vi "ITX Example.vi"() -> ()   [LabVIEW 2013]
panel:
  in  "number4":dbl=7.0
  in  "number3":dbl=5.0
  in  "number2":dbl=3.0
  in  "number1":dbl
  in  "plot2":cluster{dbl[], dbl[]}(graph)={[100000.0, 125892.54117941661, 158489.3192461114, 199526.2314968879, 251188.6431509582, 316227.7660168379, 398107.1705534969, 501187.2336272725, 630957.344480193, 794328.2347242822, 1000000.0, 1258925.411794166, 1584893.192461114, 1995262.314968879, 2511886.431509582, 3162277.66016838, 3981071.705534969, 5011872.336272725, 6309573.44480193, 7943282.347242822, 10000000.0, 12589254.117941663, 15848931.924611142, 19952623.14968883, 25118864.315095823, 31622776.60168379, 39810717.05534969, 50118723.36272725, 63095734.44801943, 79432823.47242822, 100000000.0, 125892541.17941661, 158489319.2461111, 199526231.49688828, 251188643.1509582, 316227766.01683795, 398107170.5534969, 501187233.6272715, 630957344.4801943, 794328234.7242821, 1000000000.0], [0.0604667, 0.002433367000000003, 0.02919999, 0.036766673, 0.07459995999999999, 0.058766570000000004, 0.02630003, -0.0314666, 0.03733326, -0.01006674, 0.005166649999999999, -0.013299987000000001, 0.01406666, 0.008233343, 0.008333337, -0.003000007000000001, 0.00923335, 0.009000003, 0.011999996700000001, 0.012433329, 0.0049, 0.007766663, 0.009300005, 0.0045000027, 0.006500002, 0.008566672000000001, 0.0043333317, 0.002000004, 0.005333332, 0.0038999987, 0.003166668, 0.001799999, 0.0021333357, 0.001133332, 0.004933332, 0.0021333317, 0.0025000014, 0.004033335, 0.0020666647, 0.002000003, 0.001433333]}
  in  "plot1":cluster{dbl[], dbl[]}(graph)={[100000.0, 125892.54117941661, 158489.3192461114, 199526.2314968879, 251188.6431509582, 316227.7660168379, 398107.1705534969, 501187.2336272725, 630957.344480193, 794328.2347242822, 1000000.0, 1258925.411794166, 1584893.192461114, 1995262.314968879, 2511886.431509582, 3162277.66016838, 3981071.705534969, 5011872.336272725, 6309573.44480193, 7943282.347242822, 10000000.0, 12589254.117941663, 15848931.924611142, 19952623.14968883, 25118864.315095823, 31622776.60168379, 39810717.05534969, 50118723.36272725, 63095734.44801943, 79432823.47242822, 100000000.0, 125892541.17941661, 158489319.2461111, 199526231.49688828, 251188643.1509582, 316227766.01683795, 398107170.5534969, 501187233.6272715, 630957344.4801943, 794328234.7242821, 1000000000.0], [0.002666666, 0.004400004, 0.0028333406, 0.005400007, -6.666699999999994e-05, 0.006833331, 0.001999997, 0.003966663, 0.003200001, 0.003733337, 0.0034666673, 0.007700011, 0.006166671, 0.004900002000000001, 0.004133333, 0.006633334, 0.01919998, 0.06286665999999999, 0.12583327, 0.2032, 0.2774667, 0.3839666, 0.4441999, 0.4771333, 0.5964335, 0.6360335, 0.6610668000000001, 0.6360334, 0.6508001, 0.6097, 0.5689667, 0.5584333, 0.5266666, 0.4415334, 0.39940000000000003, 0.2484999, 0.3907333, 0.2028, 0.4827999, 0.3610667, 0.3846001]}
  in  "plot0":cluster{dbl[], dbl[]}(graph)={[100000.0, 125892.54117941661, 158489.3192461114, 199526.2314968879, 251188.6431509582, 316227.7660168379, 398107.1705534969, 501187.2336272725, 630957.344480193, 794328.2347242822, 1000000.0, 1258925.411794166, 1584893.192461114, 1995262.314968879, 2511886.431509582, 3162277.66016838, 3981071.705534969, 5011872.336272725, 6309573.44480193, 7943282.347242822, 10000000.0, 12589254.117941663, 15848931.924611142, 19952623.14968883, 25118864.315095823, 31622776.60168379, 39810717.05534969, 50118723.36272725, 63095734.44801943, 79432823.47242822, 100000000.0, 125892541.17941661, 158489319.2461111, 199526231.49688828, 251188643.1509582, 316227766.01683795, 398107170.5534969, 501187233.6272715, 630957344.4801943, 794328234.7242821, 1000000000.0], [3.929161e-11, 2.28883e-11, 7.743881e-11, 1.83106e-10, 2.9793e-10, 3.948231e-10, 4.566212e-10, 4.592915e-10, 4.261035e-10, 4.1885560000000003e-10, 3.776569e-10, 4.1008169999999997e-10, 3.9406009999999996e-10, 3.677387e-10, 3.864308e-10, 4.043599e-10, 4.2495899999999994e-10, 4.837062e-10, 4.768397e-10, 4.913361e-10, 4.779835e-10, 4.226704e-10, 3.98256e-10, 6.107368e-10, 8.262671999999999e-10, 1.922619e-09, 1.959242e-09, 1.733406e-09, 1.485832e-09, 1.0738448e-09, 1.396568e-09, 2.188124e-09, 3.49428e-10, 2.4109e-10, 3.1395149999999995e-10, 2.441421e-10, 8.049056999999999e-11, 4.3487779999999995e-11, 9.269760999999999e-11, 2.136242e-11, 1.90736e-11]}
  in  "Notes":string="date and time are AUTOMATICALLY saved!\nwrite your experiment notes here"
  in  "path":path=path "C:/Users/voodoo.SEAGATE/Desktop/datatest"
  in  "filename":string="datatest"
  in  "wavenames (.Vx, etc)":string[](array[string])=["plot0", "plot1", "plot2", "number1", "number2", "number3", "number4"]
  # "give everything you are saving a name,\nor else you will become confused!"
  # "\"basic\" data format is XY graph:"
  # "\"numbers\" can be saved too:"
  # "just do this to make \"XY graphs\" out of them:"
  # "make array of graphs\nto save them all:"
  # "- set path to folder\n- set base filename\n   (up to 999,999 files with same base name \n    an be written in one folder)\n- type some comments"
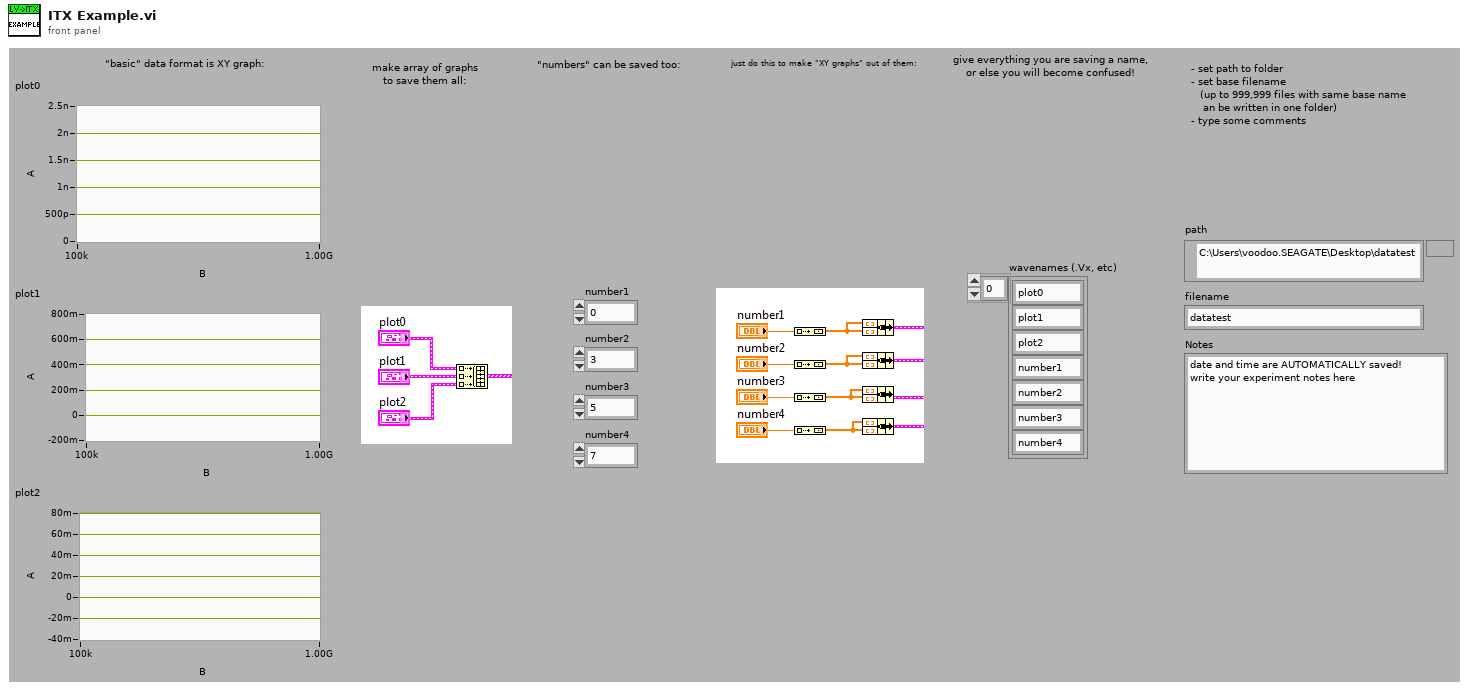
[diagram p1: front panel]
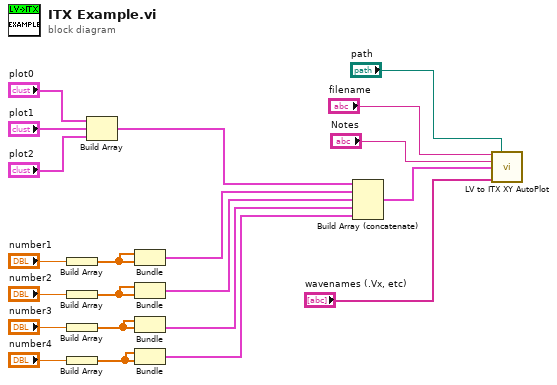
[diagram p0: block diagram]
diagram:
  n1 = Build Array("number1") -> (w15:dbl[])
  n2 = Build Array("number2") -> (w11:dbl[])
  n3 = Build Array("number3") -> (w10:dbl[])
  n4 = Build Array("number4") -> (w9:dbl[])
  n5 = Build Array("plot0", "plot1", "plot2") -> (w1:cluster{dbl[], dbl[]}[])
  n6 = Bundle(w15, w15) -> (w8:cluster{dbl[], dbl[]})  [unwired: 1 in]
  n7 = Bundle(w11, w11) -> (w7:cluster{dbl[], dbl[]})  [unwired: 1 in]
  n8 = Bundle(w10, w10) -> (w6:cluster{dbl[], dbl[]})  [unwired: 1 in]
  n9 = Bundle(w9, w9) -> (w5:cluster{dbl[], dbl[]})  [unwired: 1 in]
  n10 = Build Array (concatenate)(w1, w8, w7, w6, w5) -> (w21:cluster{dbl[], dbl[]}[])
  n11 = call "LV to ITX XY AutoPlot.vi"("filename"="filename", "path"="path", "Notes"="Notes", "XY Array"=w21, "wavenames (.Vx, etc)"="wavenames (.Vx, etc)") -> ()  [unwired: 10 in, 1 out]
